vi "Move Snake.vi"(8 "error in (no error)":errorcluster, 11 "Game Data in":T1) -> (0 "error out":errorcluster, 3 "Game Data out":T1)   [LabVIEW 2025]
uses:
  Game Data.ctl
  Bullet Data.ctl
  Game State.ctl
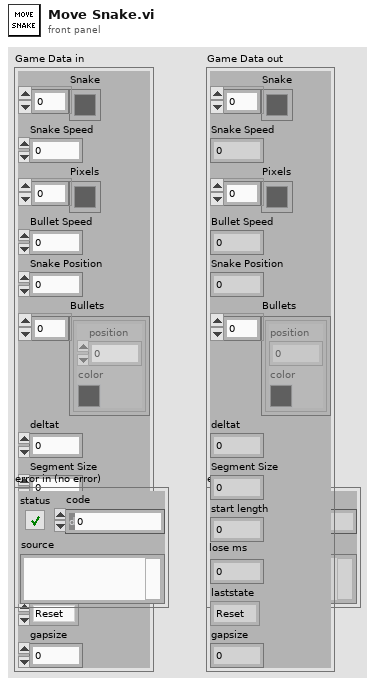
[diagram p1: front panel]
types:
  T1 = typedef "Game Data.ctl" = cluster{"Snake":u32[], "Snake Speed":dbl, "Pixels":u32[], "Bullet Speed":dbl, "Snake Position":dbl, "Bullets":T2[], "deltat":dbl, "Segment Size":dbl, "start length":u32, "lose ms":u32, "laststate":T3, "gapsize":i32}
  T2 = typedef "Bullet Data.ctl" = cluster{"position":dbl, "color":u32}
  T3 = typedef "Game State.ctl" = enum16{"Reset", "Idle", "Start", "Playing", "Win", "Lose"}
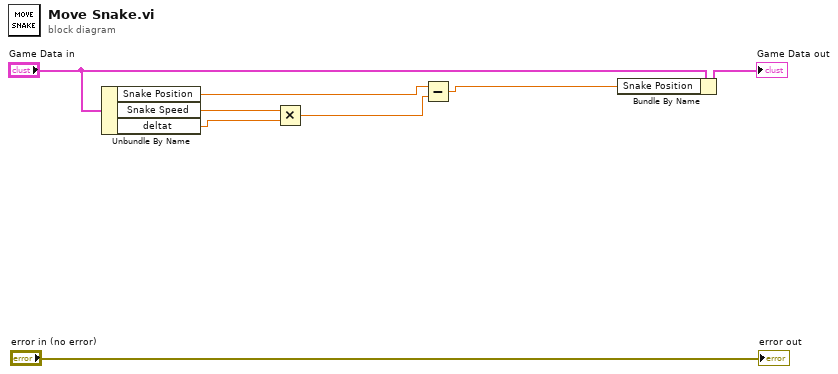
[diagram p0: block diagram]
diagram:
  n1 = Unbundle By Name("Game Data in") -> ("Snake Position"=w5:dbl, "Snake Speed"=w3:dbl, "deltat"=w1:dbl)
  n2 = Multiply(x=w3, y=w1) -> (x*y=w2:dbl)
  n3 = Subtract(x=w5, y=w2) -> (x-y=w4:dbl)
  n4 = Bundle By Name(cluster="Game Data in", "Snake Position"=w4) -> (→"Game Data out":T1)
  "error out" <- "error in (no error)"
